vi "Wait.Gui2.vi"() -> ()   [LabVIEW 2015]
uses:
  Wait.Gui.Action.ctl
panel:
  out "Knob":dbl(knob) scale=0.0..9.0 scale format="%#.1f"
  out "Numeric":dbl format="%.;%.01f %"
  in  "Color2":u32(colorbox)
  in  "Color1":u32(colorbox)=12369084
  out "_loop":i32(ring)=4
  out "status":string
  out "message":string
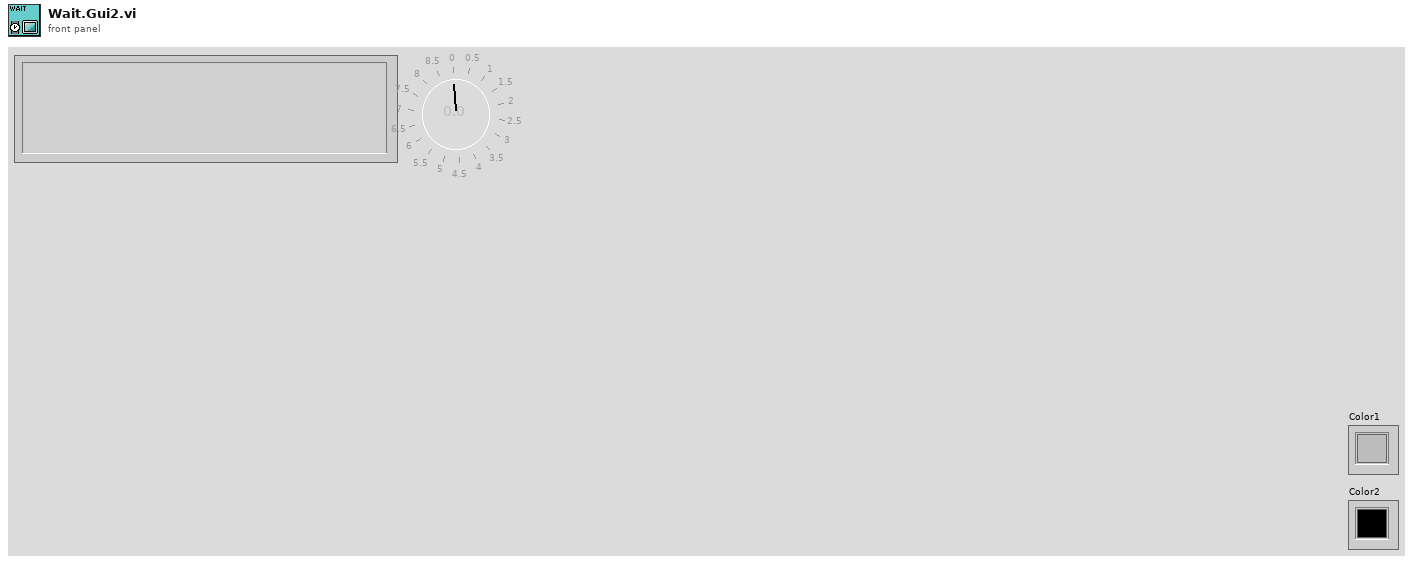
[diagram p1: front panel]
types:
  T1 = cluster{"Msg":string, "Status":string, "ProgBarSize":i32}
  T2 = enum32{"Invalid", "Standard", "Closed", "Hidden", "Minimized", "Maximized"}
  T3 = typedef "Wait.Gui.Action.ctl" = enum32{"idle", "constructor", "destructor", "--- GuiServerWait ---", "open FP", "close FP", "update msg", "update progbar"}
  T4 = typedef "LVPositionTypeDef.ctl" = cluster{"Left":i32, "Top":i32}
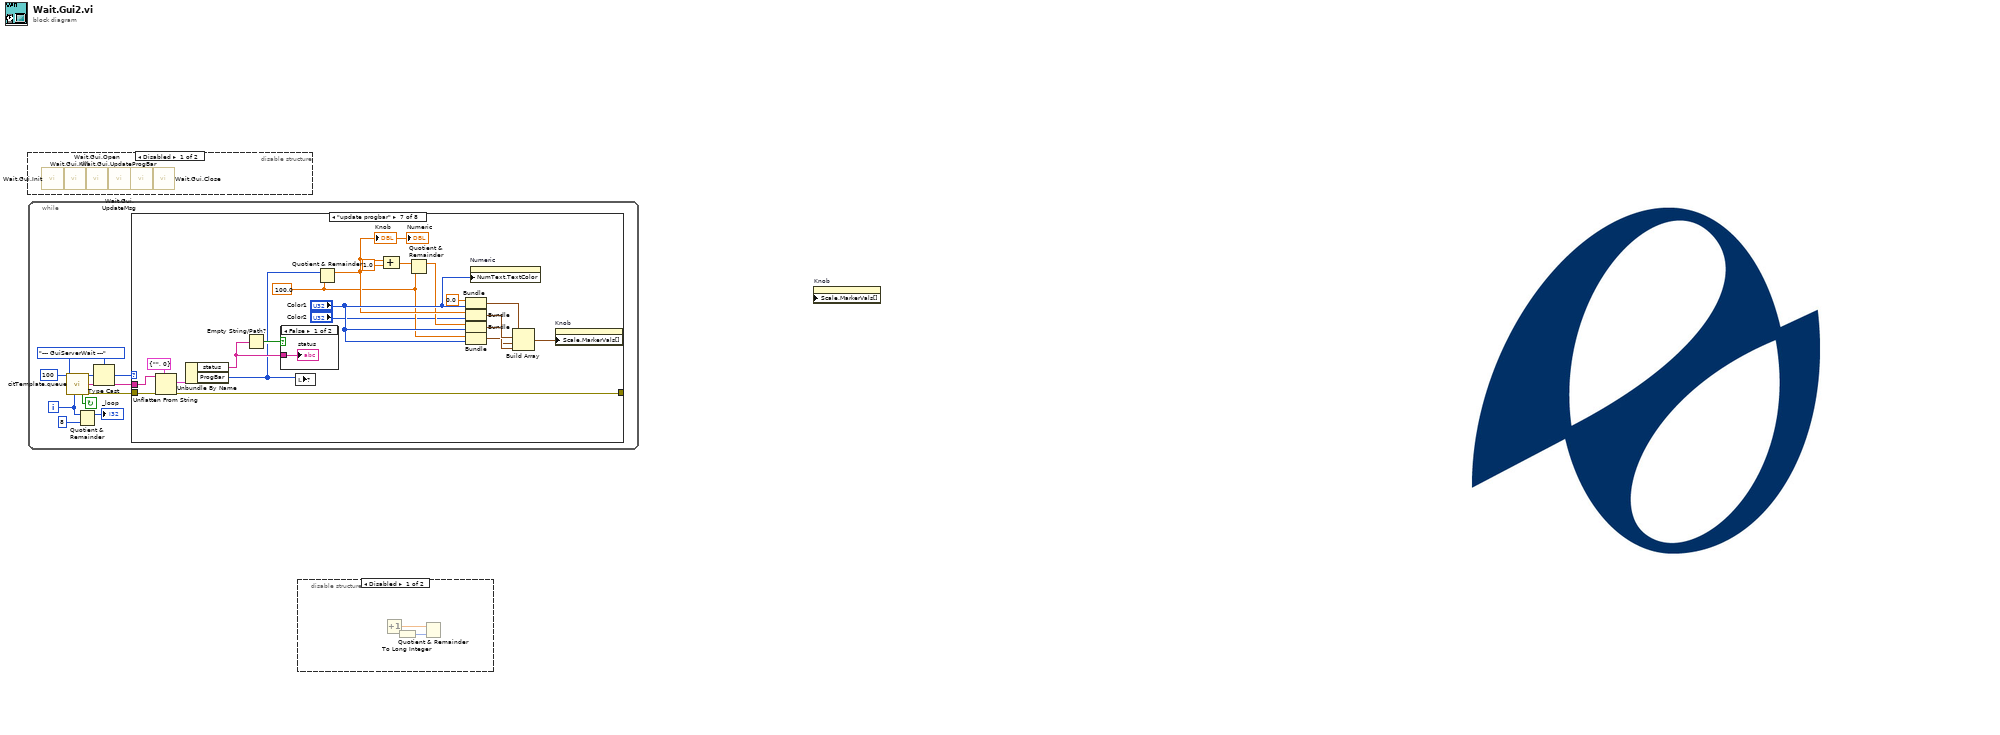
[diagram p0: block diagram]
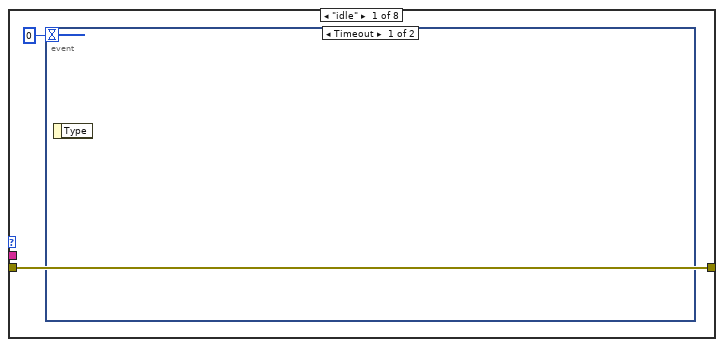
[diagram p4: hidden frame]
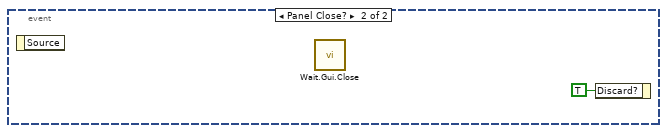
[diagram p5: hidden frame]
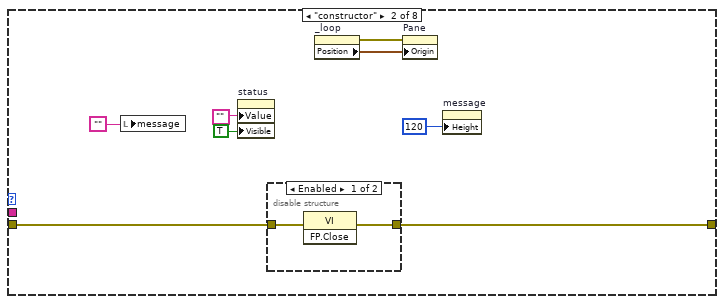
[diagram p6: hidden frame]
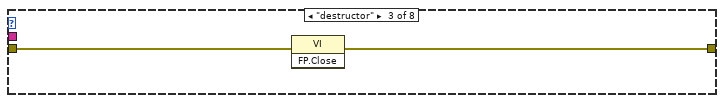
[diagram p8: hidden frame]
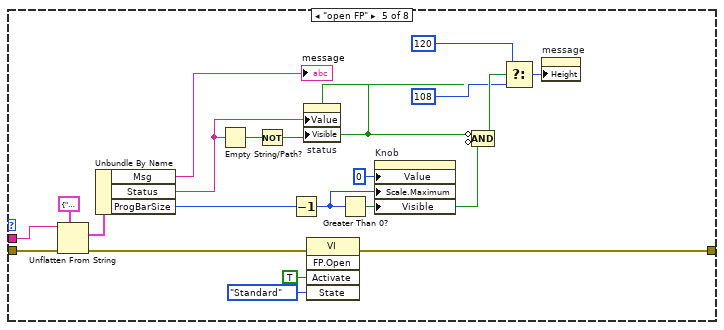
[diagram p10: hidden frame]
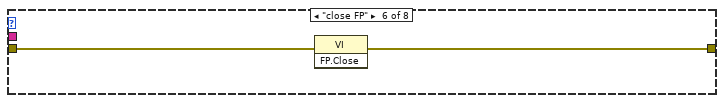
[diagram p11: hidden frame]
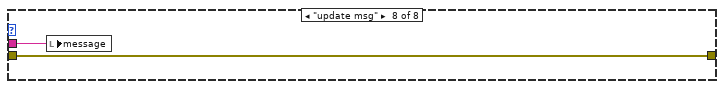
[diagram p13: hidden frame]
diagram:
  n1 = disable-structure shown="Disabled" {
    frame Disabled {
      n2 = call "Wait.Gui.Init.vi"() -> ()  [unwired: 11 in, 1 out]
      n3 = call "Wait.Gui.Kill.vi"() -> ()  [unwired: 11 in, 1 out]
      n4 = call "Wait.Gui.Open.vi"() -> ()  [unwired: 11 in, 1 out]
      n5 = call "Wait.Gui.UpdateMsg.vi"() -> ()  [unwired: 11 in, 1 out]
      n6 = call "Wait.Gui.UpdateProgBar.vi"() -> ()  [unwired: 11 in, 1 out]
      n7 = call "Wait.Gui.Close.vi"() -> ()  [unwired: 11 in, 1 out]
    }
    frame Enabled {
    }
  }
  n8 = while {
    i -> [w2]
    stop <- w4 continue-if-true
    w5 = Wait.Gui.Action."--- GuiServerWait ---" ("Action")
    n9 = call "citTemplate.queue.vi"("ms timeout (250 ms)"=100, "event enum"=w5, "iteration (-1)"=w2) -> ("event out"=w9:u32, "(flatten) data out"=w6:string, "continue"=w4:bool, "error out"=w7:errorcluster)  [unwired: 2 in, 7 out]
    n10 = Quotient & Remainder(x=w2, y=8) -> (x-y*floor(x/y)=→"_loop":i32)  [unwired: 1 out]
    n11 = Type Cast(type=w5, x=w9) -> (*(type *) &x=w8:T3)
    n12 = case shown="\"update progbar\"" w8 {
      tunnel: w7 -> [w11 w19 w25 w26 w44 w48 w69 w71]
      tunnel: w6 -> [_ _ _ _ w41 _ w68 w72]
      tunnel: [w11 w18 w24 w26 w43 w47 w67 w71] -> _
      frame "idle" {
        n13 = event shown="[0] Timeout" {
          selector: _ -> [_ _]
          dyn-events: _ -> [_ _]
          timeout: 0 -> [_ _]
          event Timeout {
            n14 = event-data() -> ()  [unwired: 1 in, 1 out]
          }
          event Panel Close? {
            n15 = event-data() -> ()  [unwired: 1 in, 1 out]
            n16 = call "Wait.Gui.Close.vi"() -> ()  [unwired: 11 in, 1 out]
            n17 = event-data("Discard?"=TRUE) -> ()  [unwired: 1 in, 1 out]
          }
        }
      }
      frame "constructor" {
        n18 = local write "message"("") -> ()
        n19 = property on="status" class="Str"("Value"="", "Visible"=TRUE) -> ()  [unwired: 2 in, 2 out]
        n20 = disable-structure shown="Enabled" {
          disable-tunnel: w19 -> [w23 _]
          disable-tunnel: [w22 _] -> w18
          frame Enabled {
            n21 = invoke class="VI" method="FP.Close"(error in=w23) -> (error out=w22:errorcluster)  [unwired: 2 in, 2 out]
          }
          frame Disabled {
          }
        }
        n22 = property on="_loop" class="Ring (strict)"() -> (error out=w20:errorcluster, "Position"=w21:T4)  [unwired: 2 in, 1 out]
        n23 = property on="Pane" class="Pane"(error in=w20, "Origin"=w21) -> ()  [unwired: 1 in, 2 out]
        n24 = property on="message" class="Str"("Height"=u32 120 ("Size:Height")) -> ()  [unwired: 2 in, 2 out]
      }
      frame "destructor" {
        n25 = invoke class="VI" method="FP.Close"(error in=w25) -> (error out=w24:errorcluster)  [unwired: 2 in, 2 out]
      }
      frame "--- GuiServerWait ---" {
      }
      frame "open FP" {
        n26 = Unflatten From String(type=T1 {"Msg"="", "Status"="", "ProgBarSize"=0} ("output cluster"), binary string=w41, error in (no error)=w44) -> (value=w39:T1, error out=w42:errorcluster)  [unwired: 2 in, 1 out]
        n27 = Unbundle By Name(w39) -> ("Msg"=→"message":string, "Status"=w34:string, "ProgBarSize"=w38:i32)
        n28 = Empty String/Path?(string/path=w34) -> (empty?=w33:bool)
        n29 = Not(x=w33) -> (.not. x?=w32:bool)
        n30 = Decrement(x=w38) -> (x-1=w37:i32)
        n31 = property on="status" class="Str"("Value"=w34, "Visible"=w32) -> ()  [unwired: 2 in, 2 out]
        n32 = invoke class="VI" method="FP.Open"(error in=w42, "Activate"=TRUE ("Activate?"), "State"=T2."Standard") -> (error out=w43:errorcluster)  [unwired: 2 in, 4 out]
        n33 = Greater Than 0?(x=w37) -> (x > 0?=w31:bool)
        n34 = property on="Knob" class="Knob (strict)"("Value"=0 ("Slide"), "Scale.Maximum"=w37, "Visible"=w31) -> ()  [unwired: 2 in, 2 out]
        n35 = Compound Arithmetic op=AND(invert w32, invert w31) -> (w29:bool)
        n36 = Select(t=u32 120 ("Size:Height"), s=w29, f=u32 108 ("Size:Height")) -> (s? t:f=w30:u32)
        n37 = property on="message" class="Str"("Height"=w30) -> ()  [unwired: 2 in, 2 out]
      }
      frame "close FP" {
        n38 = invoke class="VI" method="FP.Close"(error in=w48) -> (error out=w47:errorcluster)  [unwired: 2 in, 2 out]
      }
      frame "update progbar" {
        w60 = 100.0 ("y")
        n39 = Unflatten From String(type=cluster{"status":string, "ProgBar":i32} {"status"="", "ProgBar"=0} ("output cluster"), binary string=w68, error in (no error)=w69) -> (value=w65:cluster{"status":string, "ProgBar":i32}, error out=w67:errorcluster)  [unwired: 2 in, 1 out]
        n40 = Unbundle By Name(w65) -> ("status"=w63:string, "ProgBar"=w49:i32)
        n41 = Empty String/Path?(string/path=w63) -> (empty?=w64:bool)
        n42 = case shown="False" w64 {
          tunnel: w63 -> [w70 _]
          frame False {
            "status" <- w70
          }
          frame True {
          }
        }
        n43 = local write item#-1(w49) -> ()
        n44 = Quotient & Remainder(x=w49, y=w60) -> (x-y*floor(x/y)=w61:dbl)  [unwired: 1 out]
        "Numeric" <- w61
        "Knob" <- w61
        n45 = Compound Arithmetic op=ADD(w61, 1.0 ("value")) -> (w58:dbl)
        n46 = Quotient & Remainder(x=w58, y=w60) -> (x-y*floor(x/y)=w59:dbl)  [unwired: 1 out]
        n47 = Bundle(0.0, "Color1"="Color1") -> (w51:cluster{dbl, "Color1":u32})  [unwired: 1 in]
        n48 = Bundle(w61, "Color2"="Color2") -> (w54:cluster{dbl, "Color2":u32})  [unwired: 1 in]
        n49 = Bundle(w59, "Color1"="Color1") -> (w52:cluster{dbl, "Color1":u32})  [unwired: 1 in]
        n50 = Bundle("y"=w60, "Color1"="Color1") -> (w53:cluster{"y":dbl, "Color1":u32})  [unwired: 1 in]
        n51 = property on="Numeric" class="DigNum (strict)"("NumText.TextColor"="Color1") -> ()  [unwired: 2 in, 2 out]
        n52 = Build Array(w51, w54, w52, w53) -> (w55:cluster{"y":dbl, "Color1":u32}[])
        n53 = property on="Knob" class="Knob (strict)"("Scale.MarkerVals[]"=w55) -> ()  [unwired: 2 in, 2 out]
      }
      frame "update msg" {
        n54 = local write "message"(w72) -> ()
      }
    }
  }
  n55 = disable-structure shown="Disabled" {
    frame Disabled {
      n56 = Increment() -> (x=w74:dbl, x+1=w73:dbl)
      n57 = To Long Integer() -> (number=w75:i32, 32bit integer=w76:i32)
      n58 = Quotient & Remainder(x=w73, y=w76) -> ()  [unwired: 2 out]
    }
    frame Enabled {
    }
  }
  n59 = property on="Knob" class="Knob (strict)" props=["Scale", "MarkerVals[]"]() -> ()  [unwired: 3 in, 2 out]
